vi "Info from Source.vi"(8 "error in (no error)":errorcluster, 9 "Branch (Default)":string, 10 "Source":string, 11 "NamedPackage in":refnum<class "NamedPackage.lvclass">) -> (0 "error out":errorcluster, 2 "Package Info":T1, 3 "NamedPackage out":refnum<class "NamedPackage.lvclass">)   [LabVIEW 2020, in "GPack.lvlib" / "NamedPackage.lvclass"]
uses:
  NamedPackage.lvclass
  Package Info.ctl
  NamedPackage.lvclass/NamedPackage.ctl
  GPack File/GPack File.lvclass
  GPack.lvlib
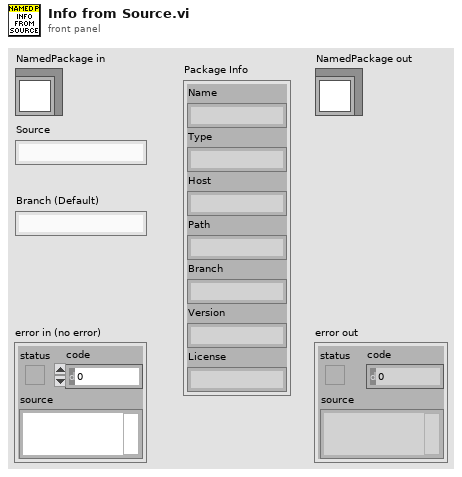
[diagram p1: front panel]
types:
  T1 = typedef "GPack.lvlib/Package Info.ctl" = cluster{"Name":string, "Type":string, "Host":string, "Path":string, "Branch":string, "Version":string, "License":string}
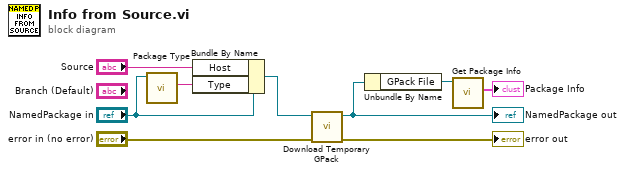
[diagram p0: block diagram]
diagram:
  n1 = call-dynamic "Package Type.vi"("NamedPackage in"="NamedPackage in") -> ("Package Type"=w2:string)  [unwired: 9 in, 1 out]
  n2 = Bundle By Name(cluster="NamedPackage in", "Host"="Source", "Type"=w2) -> (w4:refnum<class "NamedPackage.lvclass">)
  n3 = call "Download Temporary GPack.vi"("error in (no error)"="error in (no error)", "NamedPackage in"=w4) -> ("error out"=→"error out":errorcluster, "NamedPackage out"=w6:refnum<class "NamedPackage.lvclass">)  [unwired: 8 in]
  "NamedPackage out" <- w6
  n4 = Unbundle By Name(w6) -> ("GPack File"=w8:refnum<class "GPack File.lvclass">)
  n5 = call "Get Package Info.vi"("GPack File in"=w8) -> ("Package Info"=→"Package Info":T1)  [unwired: 10 in]
